vi "ENS210_WriteI2C.vi"(6 "error in (no error)":errorcluster, 8 "Bytes to Write":u8[](array[numeric]), 9 "Slave Address (7-bit)":u8) -> (0 "error out":errorcluster)   [LabVIEW 2016]
doc: "Writes data to or reads data from an Inter-Integrated Circuit (I2C) slave device through the I2C channels.\n--------------------\n\nThis Express VI is configured as follows:\n\nNode name: Pressure Sensor$\nChannel: A/I2C\nMode: Write\nSpeed: Fast mode (400 kbps)"
uses:
  <vilib>/myRIO/Instrument Drivers/Onboard IO/I2C/typedefs/I2C Reference.ctl
  <vilib>/myRIO/Common/Instrument Driver Framework/Utilities/typedefs/myRIO Generic Hardware Reference.ctl
  <vilib>/myRIO/Common/Instrument Driver Framework/Utilities/typedefs/Hardware Version Enum.ctl
  <vilib>/myRIO/Common/Instrument Driver Framework/Utilities/typedefs/myRIO v1.0 Reference.ctl
  <vilib>/myRIO/Common/Instrument Driver Framework/Utilities/typedefs/Generic FPGA Reference.ctl
  <vilib>/myRIO/Common/Instrument Driver Framework/myRIO v1.0/I2C/typedefs/I2C Channels Enum.ctl
  <vilib>/myRIO/Instrument Drivers/Onboard IO/I2C/typedefs/I2C Configuration.ctl
  <vilib>/myRIO/Instrument Drivers/Onboard IO/I2C/typedefs/I2C Transfer Rate.ctl
  <vilib>/myRIO/Instrument Drivers/Onboard IO/I2C/typedefs/I2C User Configuration.ctl
  <vilib>/myRIO/Common/Instrument Driver Framework/myRIO v1.0/I2C/vis/myRIO v1.0 Write I2C.vi
  <vilib>/Utility/error.llb/Error Cluster From Error Code.vi
  <vilib>/myRIO/Common/Instrument Driver Framework/myRIO v1.0/I2C/vis/myRIO v1.0 Configure I2C.vi
  <vilib>/myRIO/Instrument Drivers/Onboard IO/I2C/I2C.lvlib
panel:
  out "I2C Ref Out":T1={"myRIO Reference"={"myRIO Model"=enum."Unknown", "myRIO Hardware Reference"={"Generic FPGA Reference"=refnum, "Allow multiple opens"=FALSE}}, "I2C Channels Enum"=enum."Not Connected", "I2C Configuration"={"I2C Transfer Rate"=enum."Fast mode (400 kbps)"}}
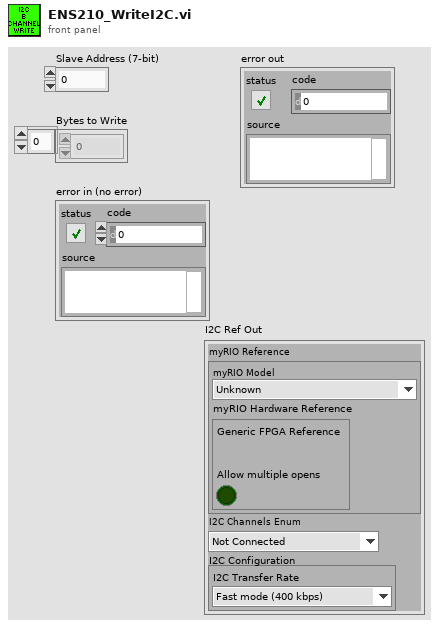
[diagram p1: front panel]
types:
  T1 = typedef "I2C.lvlib/I2C Reference.ctl" = cluster{"myRIO Reference":T2, "I2C Channels Enum":T6, "I2C Configuration":T7}
  T2 = typedef "myRIO Generic Hardware Reference.ctl" = cluster{"myRIO Model":T3, "myRIO Hardware Reference":T4}
  T3 = typedef "Hardware Version Enum.ctl" = enum16{"Unknown", "myRIO-1900", "myRIO-1950", "roboRIO", "NI ELVIS RIO CM"}
  T4 = typedef "myRIO v1.0 Reference.ctl" = cluster{"Generic FPGA Reference":T5, "Allow multiple opens":bool}
  T5 = typedef "Generic FPGA Reference.ctl" = refnum<k20>
  T6 = typedef "I2C Channels Enum.ctl" = enum16{"Not Connected", "A/I2C", "B/I2C", "I2C/I2C"}
  T7 = typedef "I2C.lvlib/I2C Configuration.ctl" = cluster{"I2C Transfer Rate":T8}
  T8 = typedef "I2C.lvlib/I2C Transfer Rate.ctl" = enum16{"Standard mode (100 kbps)", "Fast mode (400 kbps)"}
  T9 = typedef "I2C.lvlib/I2C User Configuration.ctl" = cluster{"I2C Transfer Rate":T8}
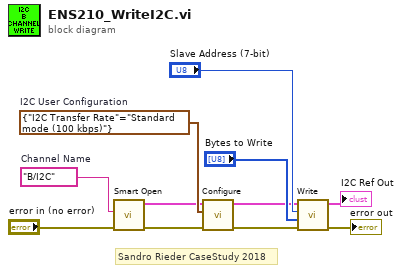
[diagram p0: block diagram]
diagram:
  w10 = T9 {"I2C Transfer Rate"=enum."Standard mode (100 kbps)"}  # I2C User Configuration
  w11 = tag "B/I2C"  # Channel Name
  # "Sandro Rieder CaseStudy 2018"
  n1 = call <vilib>:"Smart Open.vi"("error in (no error)"="error in (no error)", "Channel Name"=w11) -> ("error out"=w5:errorcluster, "I2C Ref Out"=w6:T1)  [unwired: 8 in]
  n2 = call <vilib>:"Configure.vi"("error in (no error)"=w5, "I2C User Configuration"=w10, "I2C Ref In"=w6) -> ("error out"=w3:errorcluster, "I2C Ref Out"=w4:T1)  [unwired: 7 in]
  n3 = call <vilib>:"Write.vi"("error in (no error)"=w3, "Bytes to Write"="Bytes to Write", "Slave Address (7-bit)"="Slave Address (7-bit)", "I2C Ref In"=w4) -> ("error out"=→"error out":errorcluster, "I2C Ref Out"=→"I2C Ref Out":T1)  [unwired: 6 in]
